vi "fgv_GNSS-Ntrip_param_save-load.vi"(7 "ctl":T1(ring), 8 "error in":errorcluster, 11 "file name":string) -> (0 "error out":errorcluster, 3 "open cancelled":bool caption="취소됨")   [LabVIEW 2019]
uses:
  Ctrl/cmd_common.ctl
  <vilib>/Utility/xml.llb/Write to XML File(string).vi
  <vilib>/Utility/xml.llb/Read From XML File(string).vi
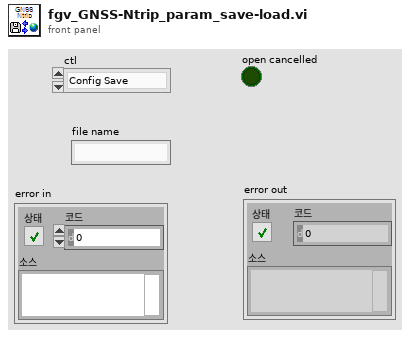
[diagram p1: front panel]
types:
  T1 = enum16{"Config Save", "Config Load", "LastRUN Save", "LastRUN Load"}
  T2 = typedef "cmd_common.ctl" = enum16{"read", "write"}
  T3 = typedef "GNSS-Ntrip config.ctl" = cluster{"Current Ntrip account":T4, "Ntrip accounts":T4[], "Mount points":u16, "Ref r size":dbl, "TMarr limit":i32, "Sel NMEA type":enum16{"$GPGSV", "$GLGSV", "$GPGGA", "$GAGSV", "$GBGSV", "$GNGLL", "$GNGGA", "$GNGSA", "$GNRMC", "$GNVTG"}, "Local Time offset":u32, "Write delay ms":u32, "GNSS Serial delay":u32, "Send Serial delay":u32, "Send Serial config":cluster{"NMEA out port":refnum<visa-resource-name>, "baud rate":u32}, "Mount point arr":string[]}
  T4 = typedef "Ntrip_Account_db.ctl" = cluster{"address":string, "port ":u16, "id":string, "pwd":string, "ref pt":string}
  T5 = typedef "gnss_config-2.ctl" = cluster{"Port":refnum<visa-resource-name>, "rate":u32}
  T6 = enum16{"open", "replace", "create", "open or create", "replace or create", "replace or create with confirmation"}
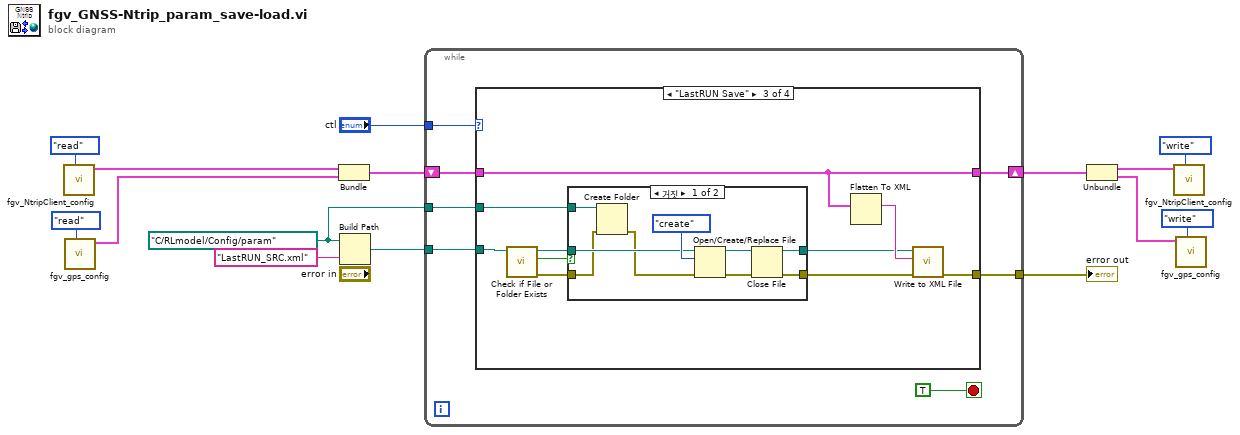
[diagram p0: block diagram]
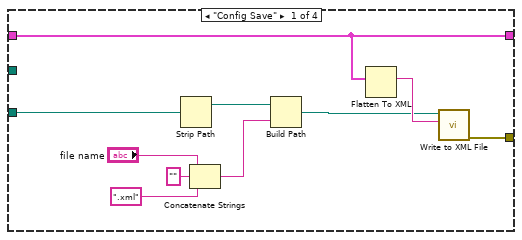
[diagram p2: hidden frame]
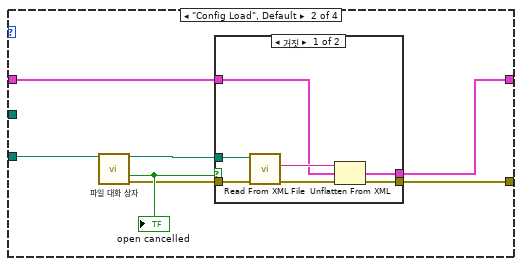
[diagram p3: hidden frame]
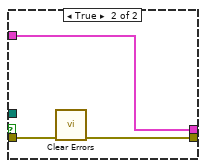
[diagram p4: hidden frame]
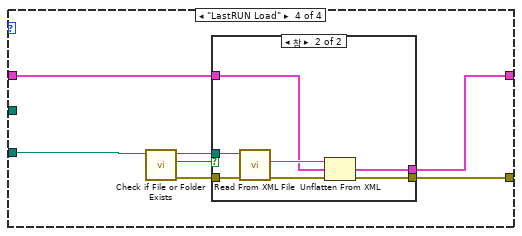
[diagram p6: hidden frame]
diagram:
  w1 = path "C:/RLmodel/Config/param" ("XML File Path")
  n1 = call "fgv_NtripClient_config.vi"("cmd"=cmd_common."read") -> ("config val out"=w10:T3)  [unwired: 10 in]
  n2 = call "fgv_gps_config.vi"("cmd"=enum16{"read", "write"}."read") -> ("GNSS cfg out"=w8:T5)  [unwired: 9 in, 1 out]
  n3 = Bundle("config val out"=w10, "GNSS cfg out"=w8) -> (w7:cluster{"config val out":T3, "GNSS cfg out":T5})  [unwired: 1 in]
  n4 = Build Path(base path=w1, name or relative path="LastRUN_SRC.xml" ("이름 또는 상대 경로")) -> (appended path=w12:path)
  n5 = while {
    tunnel: [w22] -> w15
    tunnel: "ctl" -> [w21]
    tunnel: w12 -> [w19]
    shift-right: [w18] -> w4
    shift-left: w7 -> [w20]
    tunnel: w1 -> [w16]
    stop <- TRUE stop-if-true
    n6 = case shown="\"LastRUN Save\"" w21 {
      tunnel: w20 -> [w27 w36 w53 w77]
      tunnel: w19 -> [w30 w39 w52 w71]
      tunnel: [w31 w34 w54 w75] -> w22
      tunnel: [w27 w33 w53 w76] -> w18
      tunnel: w16 -> [_ _ w50 _]
      frame "Config Save" {
        n7 = Strip Path(path=w30) -> (stripped path=w29:path)  [unwired: 1 out]
        n8 = Concatenate Strings("file name", "" ("문자열"), ".xml" ("문자열")) -> (w28:string)
        n9 = Build Path(base path=w29, name or relative path=w28) -> (appended path=w24:path)
        n10 = Flatten To XML(anything=w27) -> (xml string=w32:string)
        n11 = call-poly <vilib>:"Write to XML File.vi"("XML Input"=w32, "XML File Path"=w24) -> ("error out"=w31:errorcluster)  [unwired: 7 in, 2 out]
      }
      frame "Config Load", Default {
        n12 = call "파일 대화 상자"("start path"=w39) -> ("selected path"=w37:path, "cancelled"=w38:bool, "error out"=w35:errorcluster)  [unwired: 11 in, 1 out]
        "open cancelled" <- w38
        n13 = case shown="거짓" w38 {
          tunnel: w37 -> [w45 _]
          tunnel: w36 -> [w44 w49]
          tunnel: [w43 w49] -> w33
          tunnel: w35 -> [w41 w48]
          tunnel: [w40 w47] -> w34
          frame False {
            n14 = call-poly <vilib>:"Read From XML File.vi"("error in (no error)"=w41, "XML File Path"=w45) -> ("error out"=w42:errorcluster, "XML Elements"=w46:string)  [unwired: 7 in, 1 out]
            n15 = Unflatten From XML(xml string=w46, type=w44, error in (no error)=w42) -> (value=w43:cluster{"config val out":T3, "GNSS cfg out":T5}, error out=w40:errorcluster)
          }
          frame True {
            n16 = call <vilib>:"Clear Errors.vi"("error in (no error)"=w48) -> ("error out"=w47:errorcluster)  [unwired: 5 in, 1 out]
          }
        }
      }
      frame "LastRUN Save" {
        n17 = call <vilib>:"Check if File or Folder Exists.vi"("path"=w52) -> ("error out"=w58:errorcluster, "file or folder exists?"=w56:bool, "dup path"=w57:path)  [unwired: 8 in]
        n18 = case shown="거짓" w56 {
          tunnel: w58 -> [w61 w70]
          tunnel: w57 -> [w63 w69]
          tunnel: [w64 w70] -> w55
          tunnel: [w65 w69] -> w51
          tunnel: w50 -> [w62 _]
          frame False {
            n19 = Create Folder(path (use dialog)=w62, error in=w61) -> (error out=w60:errorcluster)  [unwired: 1 in, 2 out]
            n20 = Open/Create/Replace File(file path (use dialog)=w63, error in=w60, operation (0:open)=T6."create" ("동작(0:open)")) -> (refnum out=w66:refnum<file>, error out=w67:errorcluster)  [unwired: 3 in, 1 out]
            n21 = Close File(refnum=w66, error in=w67) -> (path=w65:path, error out=w64:errorcluster)
          }
          frame True {
          }
        }
        n22 = Flatten To XML(anything=w53) -> (xml string=w59:string)
        n23 = call-poly <vilib>:"Write to XML File.vi"("error in (no error)"=w55, "XML Input"=w59, "XML File Path"=w51) -> ("error out"=w54:errorcluster)  [unwired: 6 in, 2 out]
      }
      frame "LastRUN Load" {
        n24 = call <vilib>:"Check if File or Folder Exists.vi"("path"=w71) -> ("error out"=w72:errorcluster, "file or folder exists?"=w73:bool, "dup path"=w74:path)  [unwired: 8 in]
        n25 = case shown="참" w73 {
          tunnel: w77 -> [_ w84]
          tunnel: [_ w83] -> w76
          tunnel: [w78 w81] -> w75
          tunnel: w74 -> [_ w80]
          tunnel: w72 -> [w78 w79]
          frame False {
          }
          frame True {
            n26 = call-poly <vilib>:"Read From XML File.vi"("error in (no error)"=w79, "XML File Path"=w80) -> ("error out"=w82:errorcluster, "XML Elements"=w85:string)  [unwired: 7 in, 1 out]
            n27 = Unflatten From XML(xml string=w85, type=w84, error in (no error)=w82) -> (value=w83:cluster{"config val out":T3, "GNSS cfg out":T5}, error out=w81:errorcluster)
          }
        }
      }
    }
  }
  "error out" <- w15
  n28 = Unbundle(w4) -> ("config val out"=w3:T3, "GNSS cfg out"=w2:T5)
  n29 = call "fgv_NtripClient_config.vi"("cmd"=cmd_common."write", "config val"=w3) -> ()  [unwired: 9 in, 1 out]
  n30 = call "fgv_gps_config.vi"("cmd"=enum16{"read", "write"}."write", "GNSS cfg"=w2) -> ()  [unwired: 8 in, 2 out]
